vi "TCRL User Interface.vi"() -> ()   [LabVIEW 2021]
panel:
  out "Lamp":dbl(slide) caption="Lamp Intensity" scale=0.0..100.0
  out "Temperature":dbl(graph)=24.995992383389208
  in  "Setpoint":dbl(slide)=25.0 scale=20.0..40.0
  in  "Fan on?":bool
  in  "D":dbl=0.003
  in  "I":dbl=0.1
  in  "P":dbl=15.0
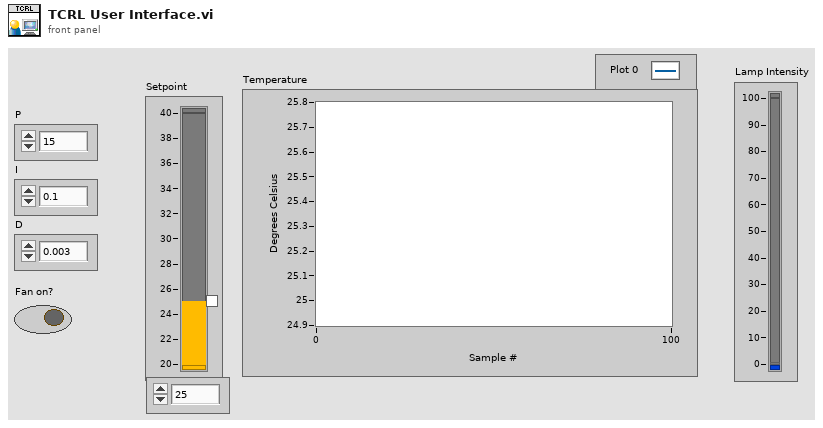
[diagram p1: front panel]
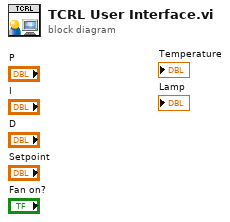
[diagram p0: block diagram]
diagram:
